vi "Init.vi"(9 "Pins":cluster{"Tx":string, "Rx":string, "UART":i8}={"Tx"="Y9", "Rx"="Y10", "UART"=0}, 11 "Python in":string="import machine, utime\n\ntx = machine.Pin('Y9', machine.Pin.OUT)\nrx = machine.Pin('Y10', machine.Pin.IN)\ntx.value(b'\\x00')\nutime.sleep_ms(500)\ntx.value(1)\n\nuart = machine.UART(3)\nuart.init(baudrate=2400, bits=8, parity=None, stop=1)\n\nuart.write(0)\n") -> (3 "Python out":string="import machine, utime\n\ntx = machine.Pin('Y9', machine.Pin.OUT)\nrx = machine.Pin('Y10', machine.Pin.IN)\ntx.value(b'\\x00')\nutime.sleep_ms(500)\ntx.value(1)\n\nuart = machine.UART(3)\nuart.init(baudrate=2400, bits=8, parity=None, stop=1)\n\nuart.write(0)\nuart.write(b'\\x40\\x23\\x9C')\n")   [LabVIEW 2016]
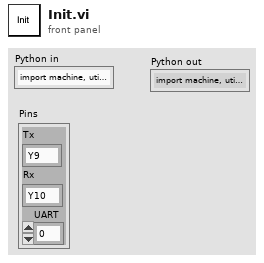
[diagram p1: front panel]
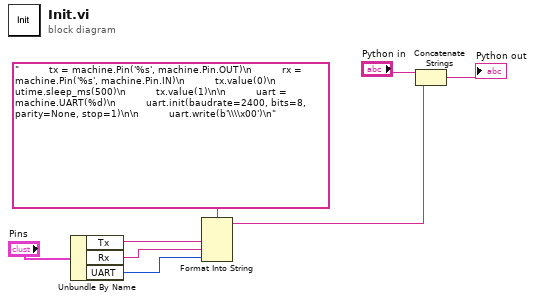
[diagram p0: block diagram]
diagram:
  n1 = Unbundle By Name("Pins") -> ("Tx"=w5:string, "Rx"=w4:string, "UART"=w3:i8)
  n2 = Format Into String(format string="          tx = machine.Pin('%s', machine.Pin.OUT)\n          rx = machine.Pin('%s', machine.Pin.IN)\n          tx.value(0)\n          utime.sleep_ms(500)\n          tx.value(1)\n\n          uart = machine.UART(%d)\n          uart.init(baudrate=2400, bits=8, parity=None, stop=1)\n\n          uart.write(b'\\\\x00')\n" ("Comment"), w5, w4, w3) -> (resulting string=w2:string)  [unwired: 2 in, 1 out]
  n3 = Concatenate Strings("Python in", w2) -> (→"Python out":string)
